vi "Read status queue.vi"(8 "error in (no error)":errorcluster, 11 "Controller in":refnum<class "Server Controller.lvclass">) -> (0 "error out":errorcluster, 2 "status queue":refnum<queue>, 3 "Controller out":refnum<class "Server Controller.lvclass">)   [LabVIEW 2026]
uses:
  Server Controller.lvclass
  C:/Users/E2013170/Documents/GitHub/Measurement-Utility-Reference/components/MAL-Framework/user.lib/Common Components/Controller/Controller.lvclass
  C:/Program Files/National Instruments/LabVIEW 2026/vi.lib/ActorFramework/Actor/Actor.lvclass
  C:/Users/E2013170/Documents/GitHub/Measurement-Utility-Reference/components/HAL-MAL-Application/Source/Framework/Server/Controller/Server Controller.lvclass
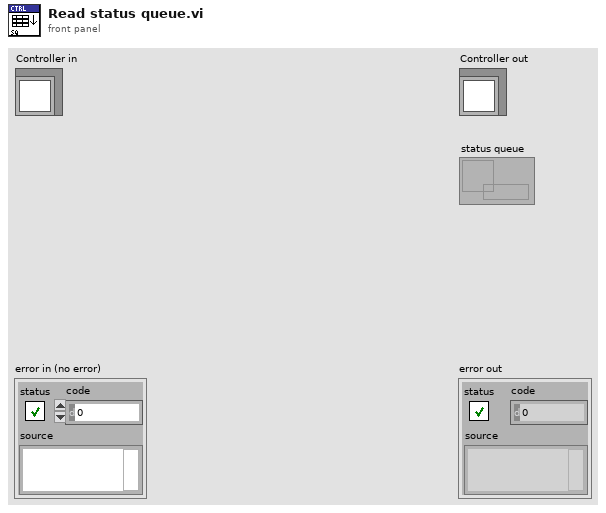
[diagram p1: front panel]
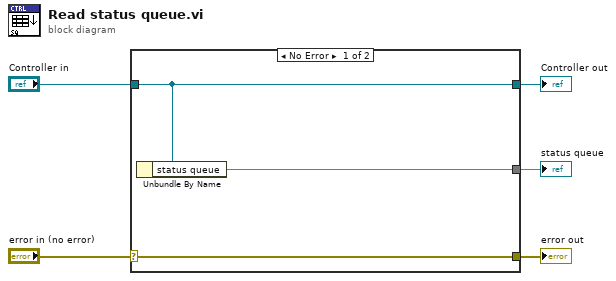
[diagram p0: block diagram]
diagram:
  n1 = case shown="No Error" "error in (no error)" {
    selector: "error in (no error)" -> [w8 w9]
    tunnel: [w8 w9] -> w4
    tunnel: [w7 w10] -> w2
    tunnel: "Controller in" -> [w7 w10]
    tunnel: [w6 _] -> w1
    frame No Error {
      n2 = Unbundle By Name(w7) -> ("status queue"=w6)
    }
    frame Error {
    }
  }
  "error out" <- w4
  "Controller out" <- w2
  "status queue" <- w1
